vi "DAQmx Create Channel (TEDS-AI-Pressure-Bridge).vi"(0 "task in":refnum<k21>, 1 "maximum value":dbl=100.0 format="%0.2f", 2 "minimum value":dbl=-100.0 format="%0.2f", 5 "physical channels":tag, 7 "name to assign":string, 9 "units":i32(ring)=15879 items=["Pascals"=10081, "psi"=15879, "bar"=15880, "From Custom Scale"=10065], 11 "error in":errorcluster, 12 "custom scale name":tag, 13 "voltage excitation source":i32(ring)=10200 items=["Internal"=10200, "External"=10167], 14 "voltage excitation value":dbl=2.5) -> (4 "task out":refnum<k21>, 15 "error out":errorcluster)   [LabVIEW 2013]
doc: "Creates channel(s) that use a Wheatstone bridge to measure pressure. You must configure the physical channel(s) with TEDS information to use this VI. NI-DAQmx scales electrical values to physical values according to that TEDS information."
uses:
  C:/Program Files (x86)/National Instruments/LabVIEW 2013/resource/objmgr/daqmx.rc
panel:
  # "input limits"
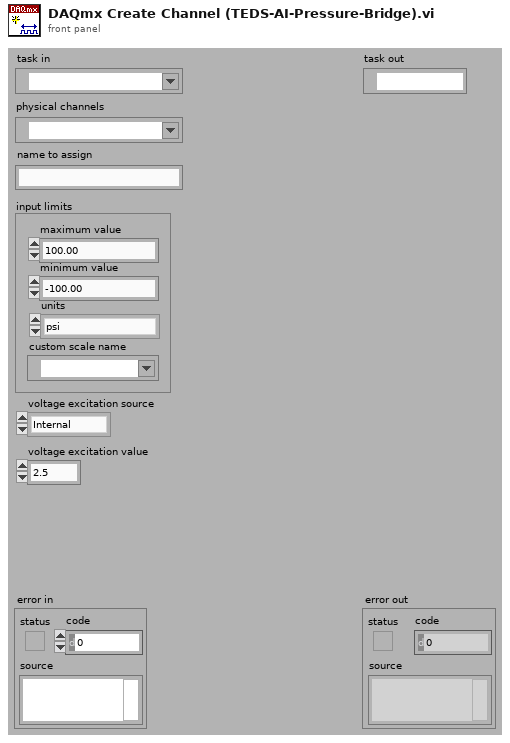
[diagram p1: front panel]
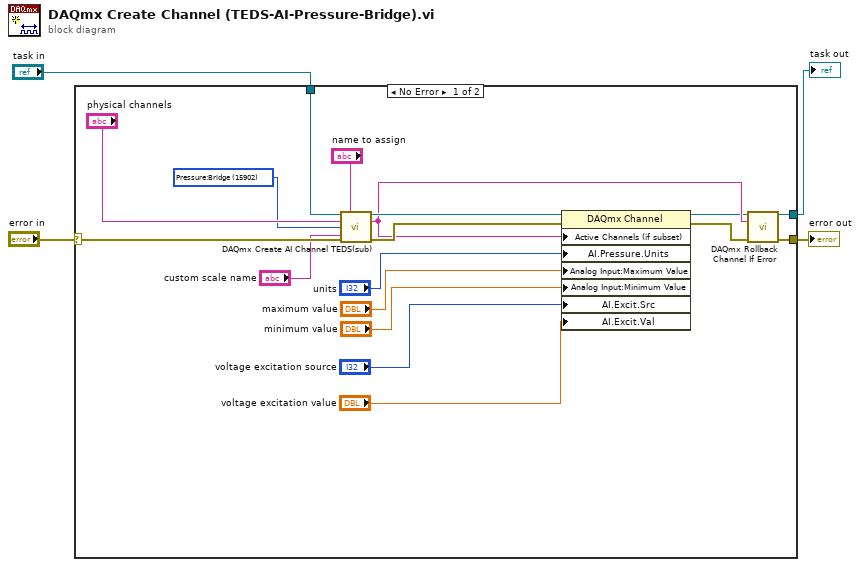
[diagram p0: block diagram]
diagram:
  n1 = case shown="No Error" "error in" {
    selector: "error in" -> [w21 w23]
    tunnel: [w13 w23] -> w4
    tunnel: "task in" -> [w22 w24]
    tunnel: [w12 w24] -> w1
    frame No Error {
      w6 = 15902 items=["Voltage"=10322, "Voltage RMS"=10350, "Current"=10134, "Current RMS"=10351, "More:Voltage:Custom with Excitation"=10323, "More:Bridge (V/V)"=15908, "Frequency"=10181, "Resistance"=10278, "Temperature:Thermocouple"=10303, "Temperature:Thermistor"=10302, "Temperature:RTD"=10301, "Temperature:Built-in Sensor"=10311, "Strain Gage"=10300, "Position:LVDT"=10352, "Position:RVDT"=10353, "Position:Eddy Current Proximity Probe"=14835, "Accelerometer"=10356, "Force:Bridge"=15899, "Force:IEPE Sensor"=15895, "Pressure:Bridge"=15902, "Sound Pressure:Microphone"=10354, "Torque:Bridge"=15905, "TEDS Sensor"=12531] ("AI.MeasType")
      n2 = call "DAQmx Create AI Channel TEDS(sub).vi"("task in"=w22, "virtual channel name"="name to assign", "physical channel name"="physical channels", "measurement type"=w6, "error in"=w21, "custom scale"="custom scale name") -> ("task out"=w14:refnum<k21>, "channel names"=w11:string, "error out"=w19:errorcluster)  [unwired: 7 out]
      n3 = property class="DAQmx Channel"(reference=w14, error in=w19, "Active Channels (if subset)"=w11, "AI.Pressure.Units"="units", "Analog Input:Maximum Value"="maximum value", "Analog Input:Minimum Value"="minimum value", "AI.Excit.Src"="voltage excitation source", "AI.Excit.Val"="voltage excitation value") -> (reference out=w10:refnum<k21>, error out=w9:errorcluster)
      n4 = call "DAQmx Rollback Channel If Error.vi"("task in"=w10, "channel names"=w11, "error in"=w9) -> ("task out"=w12:refnum<k21>, "error out"=w13:errorcluster)  [unwired: 11 out]
    }
    frame Error {
    }
  }
  "error out" <- w4
  "task out" <- w1
